vi "ADC SNR_Sweep - Copy.vi"(8 "error in (no error)":errorcluster, 9 "Sequence parameters":string[][](array[string])=[["Min limit", "Max limit", "Register sheet file", "Register Sheet"], ["", "", "CC2600.xls", "TX_BLE;Trim"], ["Reg write (addr;value)", "Operating frequency [Hz]", "", ""], ["NA", "2.44G", "", ""]], 10 "Run type":i32, 11 "Method parameters":T2={"Dev"={"Do not disturb DUT"=FALSE, "XOSC"=32000000.0, "Board type"="", "EM"="", "Configure tempboard"=TRUE, "Device specific info"=[], "Generic Object"=refnum}, "Method"={"Run type"=1, "Test name"="Current LPM2 4", "Comment"="", "Results folder"="", "AFC"=enum."Off", "Method name"="Current LPM2 4", "Method results"={"Excel brief report"=FALSE, "Spotfire report"=FALSE, "Starfish report"=FALSE}, "Operator"="", "Reference time"=timestamp(0 s since 1904-01-01), "AFC delay"=0.0, "Initialization"=enum."Enabled", "MD5 Sum"="", "HW addon board"=enum."None", "AFC Regsheet"="", "AFC Regfile"=path "", "dummy"=0.0}, "Inst"={"Instr"={"PS1"={"Name"="", "GPIB address"="", "VISA session"=""}, "PS2"={"Name"="", "GPIB address"="", "VISA session"=""}, "TC1"={"Name"="", "GPIB address"="", "VISA session"=""}, "TC2"={"Name"="", "GPIB address"="", "VISA session"=""}, "SA1"={"Name"="", "GPIB address"="", "VISA session"=""}, "SA2"={"Name"="", "GPIB address"="", "VISA session"=""}, "SG1"={"Name"="", "GPIB address"="", "VISA session"=""}, "SG2"={"Name"="", "GPIB address"="", "VISA session"=""}, "SG3"={"Name"="", "GPIB address"="", "VISA session"=""}, "MI1"={"Name"="", "GPIB address"="", "VISA session"=""}, "MI2"={"Name"="", "GPIB address"="", "VISA session"=""}, "SW SA"={"Name"="", "Controller addr"=""}, "SW SG"={"Name"="", "Controller addr"=""}, "MI3"={"Name"="", "GPIB address"="", "VISA session"=""}}, "Switchbox"={"RF Path"=0, "Cal compensation"=enum."TX", "Switchbox gain mode"="", "State"=enum."TX"}, "Instr to control (i.e. SA1)"="Default", "Intrument info string"=""}, "Sequence parameters"=[["Weight", "Min Limit", "Max Limit", "Register Sheet", "", "", "", "", "", "", "", "", ""], ["Vital", "", "1", "LPM2", "", "", "", "", "", "", "", "", ""], ["Resolution", "Reg write (addr;value)", "Chip mode", "Range", "", "", "", "", "", "", "", "", ""], ["u", "NA", "", "auto", "", "", "", "", "", "", "", "", ""]], "Cond"={"Temp logged"=25.0, "VDD1_PS1_6V"=-999.0, "VDD2_PS1_25V"=-999.0, "VDD4_PS2_25V"=-999.0, "VDD3_PS2_6V"=-999.0}, "Meas config"={"X-axis inner loop index"=32000000, "Y-axis outer loop index"=32000000, "X-axis"=[], "Y-axis"=[], "X-axis array req size"=32000000, "Y-axis array req size"=32000000, "Param description"=[], "Use meas clust for reporting"=FALSE, "Parameter index (page)"=0, "X-axis name"="", "Y-axis name"=""}} {"Cond"."VDD3_PS2_6V" format="%.3f"; "Cond"."VDD4_PS2_25V" format="%.3f"; "Cond"."VDD2_PS1_25V" format="%.3f"; "Cond"."VDD1_PS1_6V" format="%.3f"; "Method"."dummy" format="%.1p"; "Method"."AFC delay" format="%.1p"; "Dev"."XOSC" format="%.3p"}) -> (0 "Error Out":errorcluster[](array[cluster]), 1 "End Method Error":T2[](array[typedef]) {"Cond"."VDD3_PS2_6V" format="%.3f"; "Cond"."VDD4_PS2_25V" format="%.3f"; "Cond"."VDD2_PS1_25V" format="%.3f"; "Cond"."VDD1_PS1_6V" format="%.3f"; "Method"."dummy" format="%.1p"; "Method"."AFC delay" format="%.1p"; "Dev"."XOSC" format="%.3p"}, 2 "Short Results":string[](array[string]), 3 "Result summary":string[][](array[string])=[["Critical", "Output Power@2405 MHz", "-3", "4", "dBm"], ["Critical", "Output Power@2410 MHz", "-3", "4", "dBm"]])   [LabVIEW 2019]
doc: "[AutoDocStart]Performs crystal accuracy measurements. Measures the offset from ideal frequency. Primarily used for tuning XOSC capacitors and verifying XOSC trims.\n\nSweeping parameters: operating frequency, OSC override value and VDDR level\n\nResults: Offset frequency in ppm[AutoDocEnd]"
uses:
  User Lib/Utilities/Cluster definitions/Method input.ctl
  User Lib/Utilities/Cluster definitions/Device specific info.ctl
  User Lib/Utilities/Controls/Automatic Frequency Compensation types.ctl
  User Lib/Utilities/Controls/Method Reports.ctl
  User Lib/Utilities/Cluster definitions/Method Initialization.ctl
  User Lib/Utilities/Controls/HW addon boards.ctl
  User Lib/Utilities/Cluster definitions/Instr clust.ctl
  User Lib/Utilities/Switchbox control/SwitchBox_State._ENUMctl.ctl
  User Lib/Utilities/Cluster definitions/DUT vdd control.ctl
  User Lib/Utilities/Cluster definitions/DUT VDD4.ctl
  User Lib/Utilities/Cluster definitions/DUT VDD3.ctl
  User Lib/Utilities/Cluster definitions/DUT VDD2.ctl
  User Lib/Utilities/Cluster definitions/DUT VDD1.ctl
  User Lib/Generic chip methods/Classes/Generic_EM/Chameleon/Loki/Loki.lvclass
  69b5c8be-48d6-4f50-bcce-2a9f07fdba1a.vi
  1131283d-b54a-4ae3-ad67-71ff8f51acfe.vi
  3aacce8f-890b-4d9f-8ed2-28f84894822b.vi
  b456e919-2776-4fbb-a2ba-e4feed106c64.vi
  <vilib>/Utility/error.llb/Clear Errors.vi
  User Lib/Generic chip methods/Classes/Generic_EM/Chameleon/65nm.lvclass
  C:/Kharon/User Lib/Generic chip methods/Classes/Generic_EM/Generic_EM/Generic_EM.lvclass
  User Lib/Generic chip methods/board_to_chip_type.vi
  User Lib/Generic chip methods/Classes/Get_Class_init.vi
  User Lib/Generic chip methods/Classes/Generic_EM/Generic_EM/Generic_EM.lvclass
panel:
  out "Output Response [All DUTs] 7":u32[][](array[numeric])
  out "Dynamic Parameters 4":T1={"SNR"=nan, "SNRD"=nan, "THD"=nan, "ENOB (SNRD)"=nan, "SFDR"=nan, "ENOB (SNR)"=nan, "Noise Power"=nan, "Signal power"=nan} {"Signal power" format="%.6f"; "Noise Power" format="%.2f"; "ENOB (SNR)" format="%.2f"; "SFDR" format="%.2f"; "ENOB (SNRD)" format="%.2f"; "THD" format="%.2f"; "SNRD" format="%.2f"; "SNR" format="%.2f"}
  out "detected Throughput":dbl=200065.4236150998
  out "Output Response [All DUTs] 6":u32[][](array[numeric])
  out "Dynamic Parameters 3":T1={"SNR"=nan, "SNRD"=nan, "THD"=nan, "ENOB (SNRD)"=nan, "SFDR"=nan, "ENOB (SNR)"=nan, "Noise Power"=nan, "Signal power"=nan} {"Signal power" format="%.6f"; "Noise Power" format="%.2f"; "ENOB (SNR)" format="%.2f"; "SFDR" format="%.2f"; "ENOB (SNRD)" format="%.2f"; "THD" format="%.2f"; "SNRD" format="%.2f"; "SNR" format="%.2f"}
  out "detected Throughput":dbl=200065.4236150998
  out "Output Response [All DUTs] 5":u32[][](array[numeric])
  out "Dynamic Parameters 2":T1={"SNR"=nan, "SNRD"=nan, "THD"=nan, "ENOB (SNRD)"=nan, "SFDR"=nan, "ENOB (SNR)"=nan, "Noise Power"=nan, "Signal power"=nan} {"Signal power" format="%.6f"; "Noise Power" format="%.2f"; "ENOB (SNR)" format="%.2f"; "SFDR" format="%.2f"; "ENOB (SNRD)" format="%.2f"; "THD" format="%.2f"; "SNRD" format="%.2f"; "SNR" format="%.2f"}
  out "detected Throughput":dbl=200065.4236150998
  out "detected Throughput":dbl=200065.4236150998
  out "Dynamic Parameters":T1={"SNR"=nan, "SNRD"=nan, "THD"=nan, "ENOB (SNRD)"=nan, "SFDR"=nan, "ENOB (SNR)"=nan, "Noise Power"=nan, "Signal power"=nan} {"Signal power" format="%.6f"; "Noise Power" format="%.2f"; "ENOB (SNR)" format="%.2f"; "SFDR" format="%.2f"; "ENOB (SNRD)" format="%.2f"; "THD" format="%.2f"; "SNRD" format="%.2f"; "SNR" format="%.2f"}
  out "Output Response [All DUTs] 4":u32[][](array[numeric])
  in  "Tab Control":T10(tab)
  # "°C"
  # "°C"
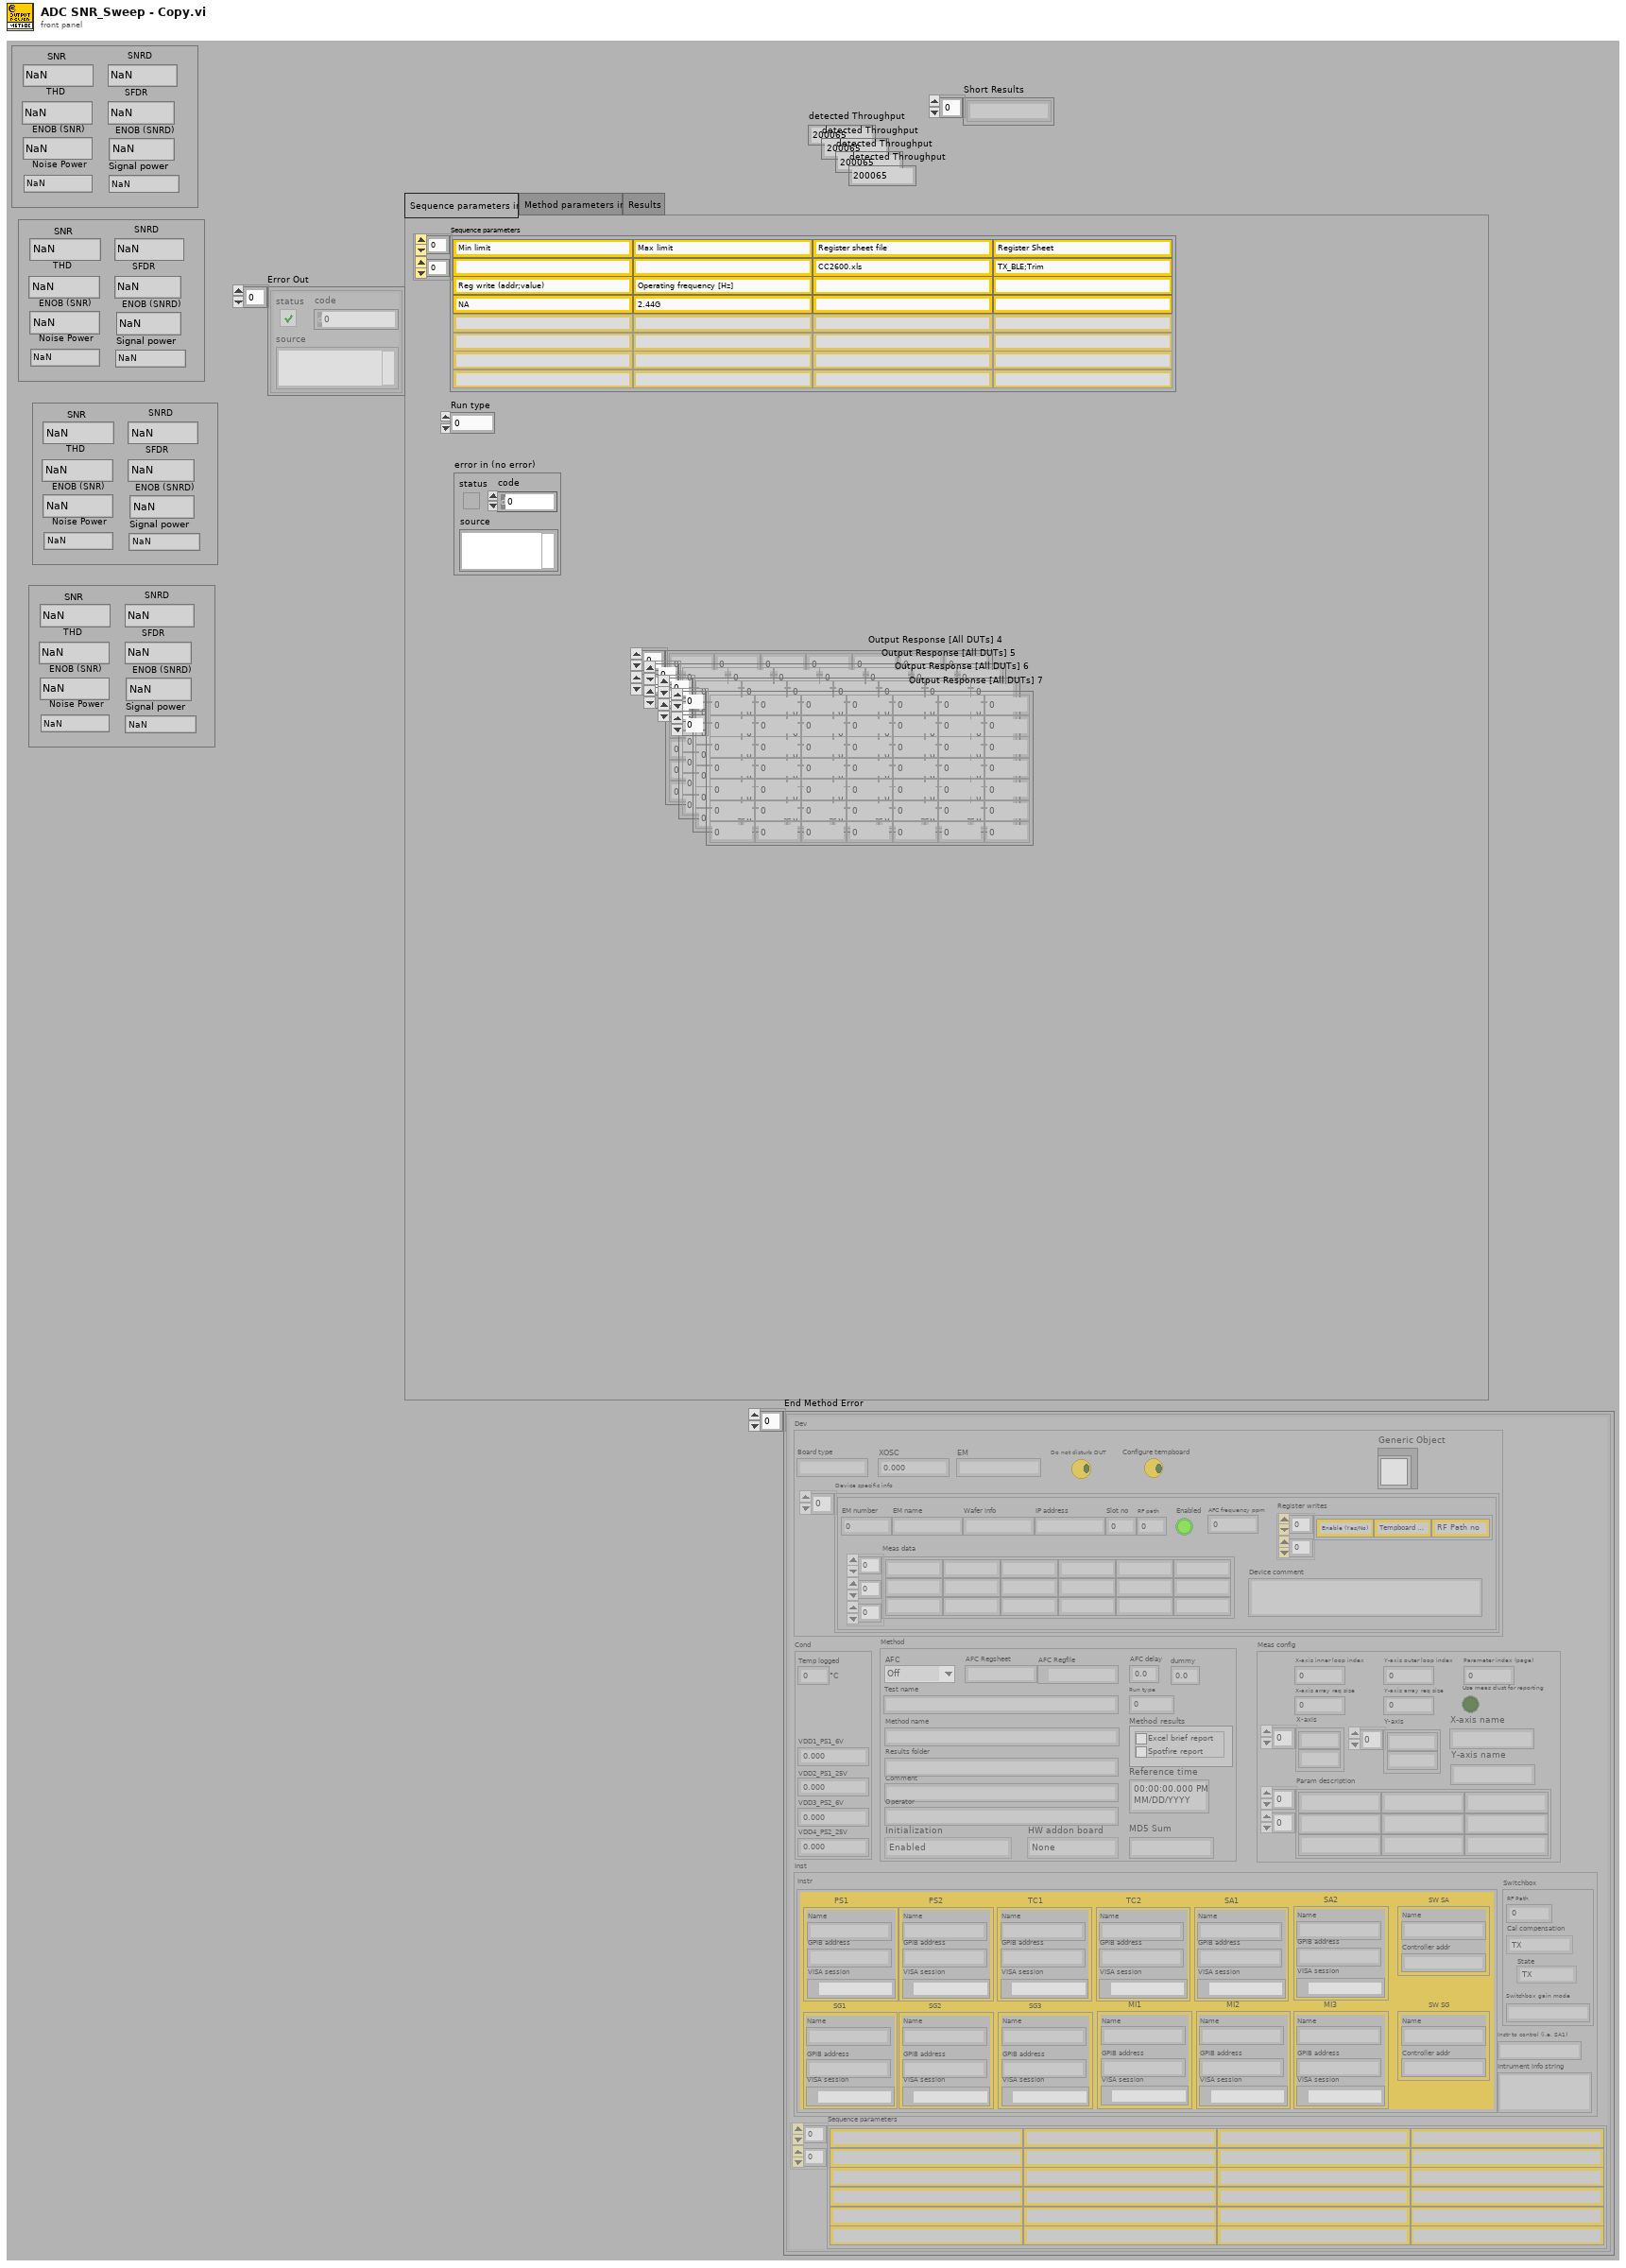
[diagram p1: front panel]
types:
  T1 = cluster{"SNR":dbl, "SNRD":dbl, "THD":dbl, "ENOB (SNRD)":dbl, "SFDR":dbl, "ENOB (SNR)":dbl, "Noise Power":dbl, "Signal power":dbl}
  T2 = typedef "Method input.ctl" = cluster{"Dev":cluster{"Do not disturb DUT":bool, "XOSC":dbl, "Board type":string, "EM":string, "Configure tempboard":bool, "Device specific info":T3[], "Generic Object":refnum<class>}, "Method":cluster{"Run type":i32, "Test name":string, "Comment":string, "Results folder":string, "AFC":T4, "Method name":string, "Method results":T5, "Operator":string, "Reference time":timestamp, "AFC delay":dbl, "Initialization":T6, "MD5 Sum":string, "HW addon board":T7, "AFC Regsheet":string, "AFC Regfile":path, "dummy":dbl}, "Inst":T8, "Sequence parameters":string[][], "Cond":cluster{"Temp logged":dbl, "VDD1_PS1_6V":dbl, "VDD2_PS1_25V":dbl, "VDD4_PS2_25V":dbl, "VDD3_PS2_6V":dbl}, "Meas config":cluster{"X-axis inner loop index":i32, "Y-axis outer loop index":i32, "X-axis":string[], "Y-axis":string[], "X-axis array req size":i32, "Y-axis array req size":i32, "Param description":string[][], "Use meas clust for reporting":bool, "Parameter index (page)":i32, "X-axis name":string, "Y-axis name":string}}
  T3 = typedef "Device specific info.ctl" = cluster{"EM number":u8, "IP address":string, "Enabled":bool, "Slot no":u8, "RF path":u8, "EM name":string, "Wafer info":string, "AFC frequency ppm":dbl, "Register writes":string[][], "Meas data":string[][][], "Device comment":string}
  T4 = typedef "Automatic Frequency Compensation types.ctl" = enum16{"Off", "Compensate Instrument frequency", "Compensate DUT frequency", "Predictive - Compensate Instrument frequency", "Predictive - Compensate DUT frequency", "Do not skip re-init - Compensate Instrument frequency", "Do not skip re-init - Compensate DUT frequency"}
  T5 = typedef "Method Reports.ctl" = cluster{"Excel brief report":bool, "Spotfire report":bool, "Starfish report":bool}
  T6 = typedef "Method Initialization.ctl" = enum16{"Enabled", "Skip Instr and Device Init", "Enabled with Separate Flash", "Set PS, Device Init and Skip Instr Init", "Skip Device Init"}
  T7 = typedef "HW addon boards.ctl" = enum16{"None", "Current meas 5EM", "Stresstest 10EM"}
  T8 = typedef "Instr clust.ctl" = cluster{"Instr":cluster{"PS1":cluster{"Name":string, "GPIB address":string, "VISA session":refnum<visa-resource-name>}, "PS2":cluster{"Name":string, "GPIB address":string, "VISA session":refnum<visa-resource-name>}, "TC1":cluster{"Name":string, "GPIB address":string, "VISA session":refnum<visa-resource-name>}, "TC2":cluster{"Name":string, "GPIB address":string, "VISA session":refnum<visa-resource-name>}, "SA1":cluster{"Name":string, "GPIB address":string, "VISA session":refnum<visa-resource-name>}, "SA2":cluster{"Name":string, "GPIB address":string, "VISA session":refnum<visa-resource-name>}, "SG1":cluster{"Name":string, "GPIB address":string, "VISA session":refnum<visa-resource-name>}, "SG2":cluster{"Name":string, "GPIB address":string, "VISA session":refnum<visa-resource-name>}, "SG3":cluster{"Name":string, "GPIB address":string, "VISA session":refnum<visa-resource-name>}, "MI1":cluster{"Name":string, "GPIB address":string, "VISA session":refnum<visa-resource-name>}, "MI2":cluster{"Name":string, "GPIB address":string, "VISA session":refnum<visa-resource-name>}, "SW SA":cluster{"Name":string, "Controller addr":string}, "SW SG":cluster{"Name":string, "Controller addr":string}, "MI3":cluster{"Name":string, "GPIB address":string, "VISA session":refnum<visa-resource-name>}}, "Switchbox":cluster{"RF Path":i32, "Cal compensation":enum16{"TX", "RX", "Interferer", "No compensation", "Interferer2"}, "Switchbox gain mode":string, "State":T9}, "Instr to control (i.e. SA1)":string, "Intrument info string":string}
  T9 = typedef "SwitchBox_State._ENUMctl.ctl" = enum16{"TX", "RX", "SP:TX", "SP:RX", "SW:TX", "SW:RX"}
  T10 = enum32{"Sequence parameters in", "Method parameters in", "Results"}
  T11 = typedef "DUT vdd control.ctl" = cluster{"VDD4 config":T12, "VDD3 config":T13, "VDD2 config":T14, "VDD1 config":T15}
  T12 = typedef "DUT VDD4.ctl" = u16
  T13 = typedef "DUT VDD3.ctl" = u16
  T14 = typedef "DUT VDD2.ctl" = u16
  T15 = typedef "DUT VDD1.ctl" = u16
  T16 = cluster{"Fundamental Frequency":dbl, "Sampling Frequncy":dbl, "No of Harmonics":u8, "Window":enum16{"None ", "Hanning", "Hamming", "Blackman-Harris", "Exact Blackman", "Blackman", "Flat Top", "4 Term B-Harris ", "7 Term B-Harris"}, "Blackman (fundamental power) bins)":dbl}
  T17 = enum32{"NI Card Settings", "Memory Read Setting", "DC Capture", "ADC Ramp", "ADC Sine", "SNR", "Cap Calibration"}
  T18 = enum32{"Read from Memory", "Read .dat file", "NI Card Capture", "None"}
  T19 = typedef "TFW ResponseData.ctl" = cluster{"errorCode":u32, "executionTime":u32, "processedCmdWord":u32, "responsePar":u32[], "actionCode":u32, "cmdStatus":u16}
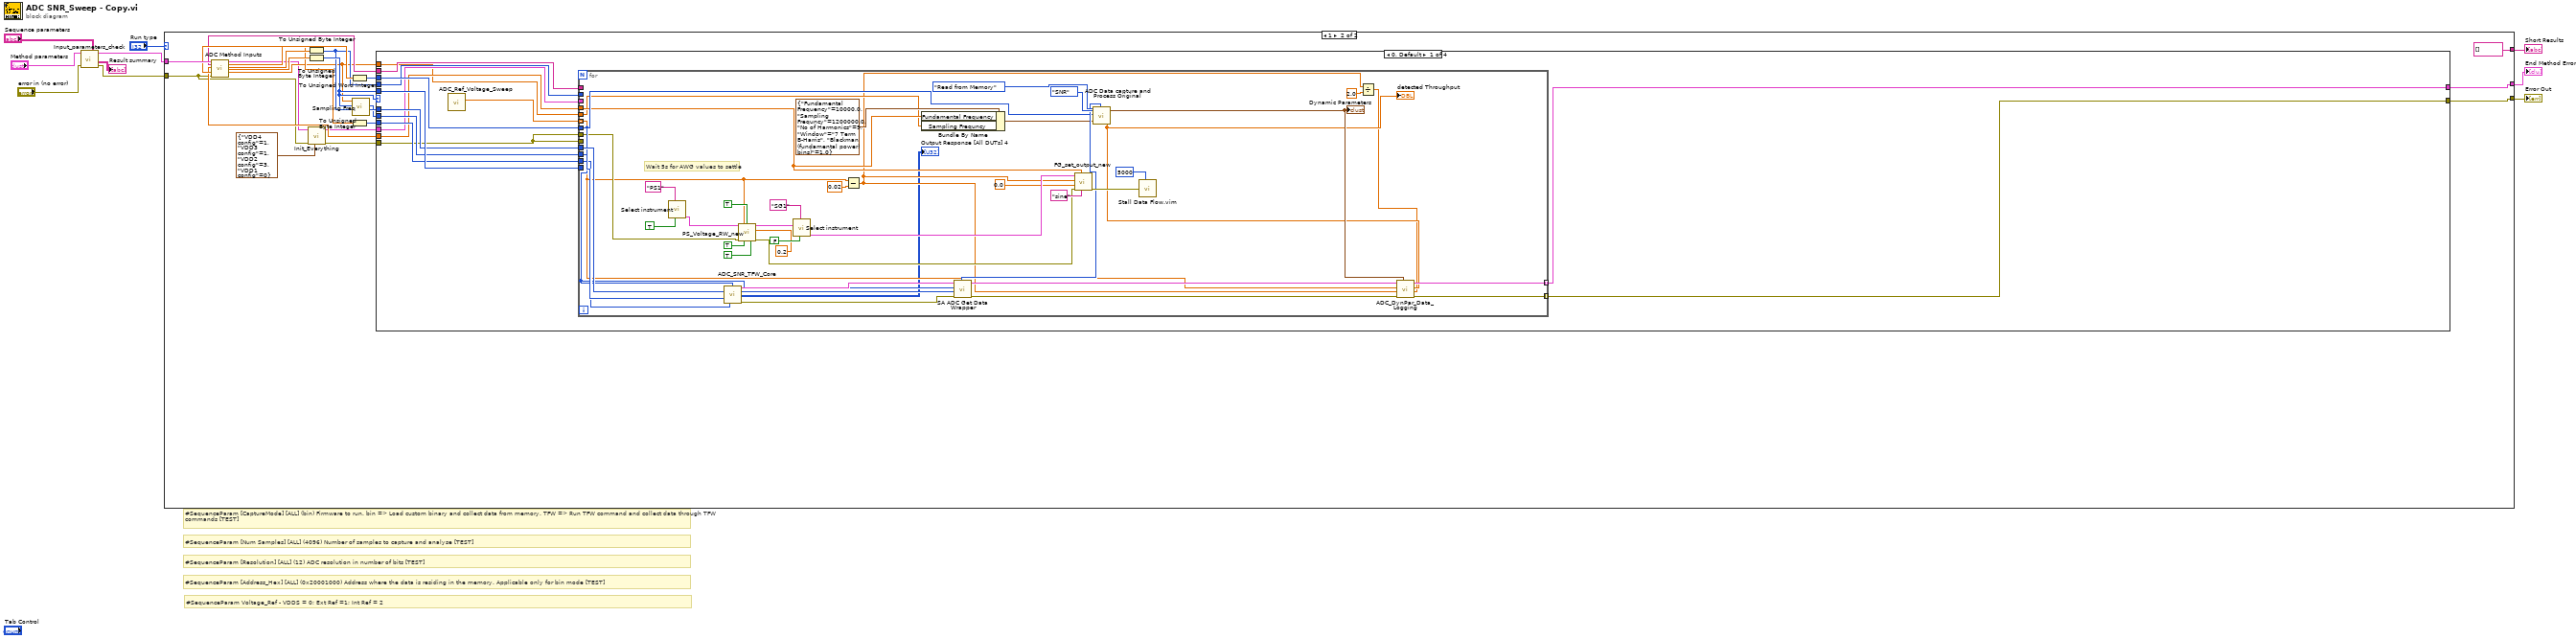
[diagram p0: block diagram]
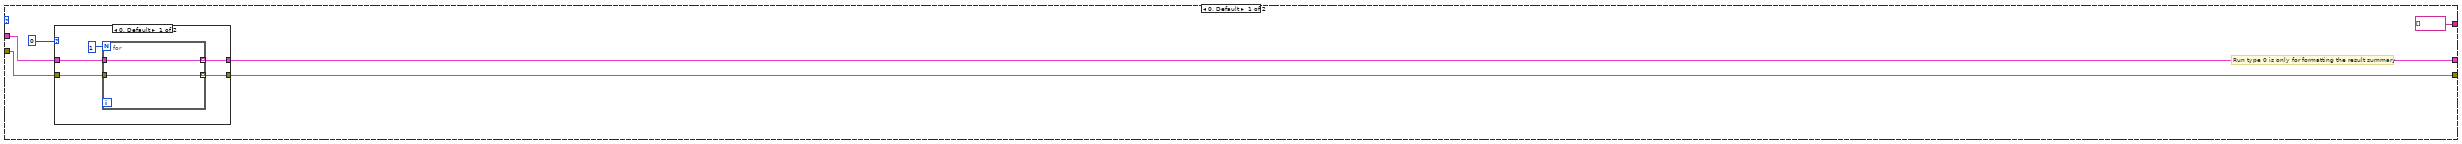
[diagram p2: hidden frame]
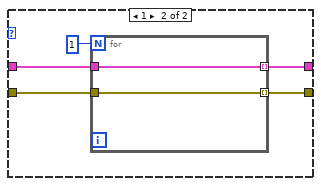
[diagram p3: hidden frame]
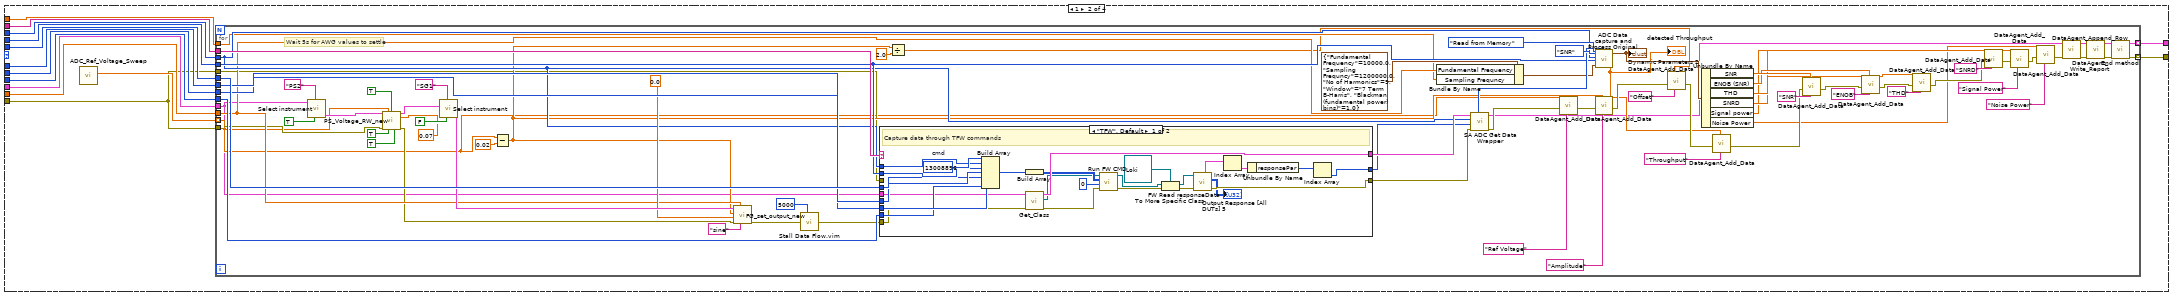
[diagram p4: hidden frame]
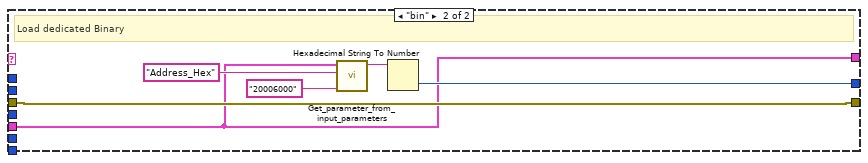
[diagram p5: hidden frame]
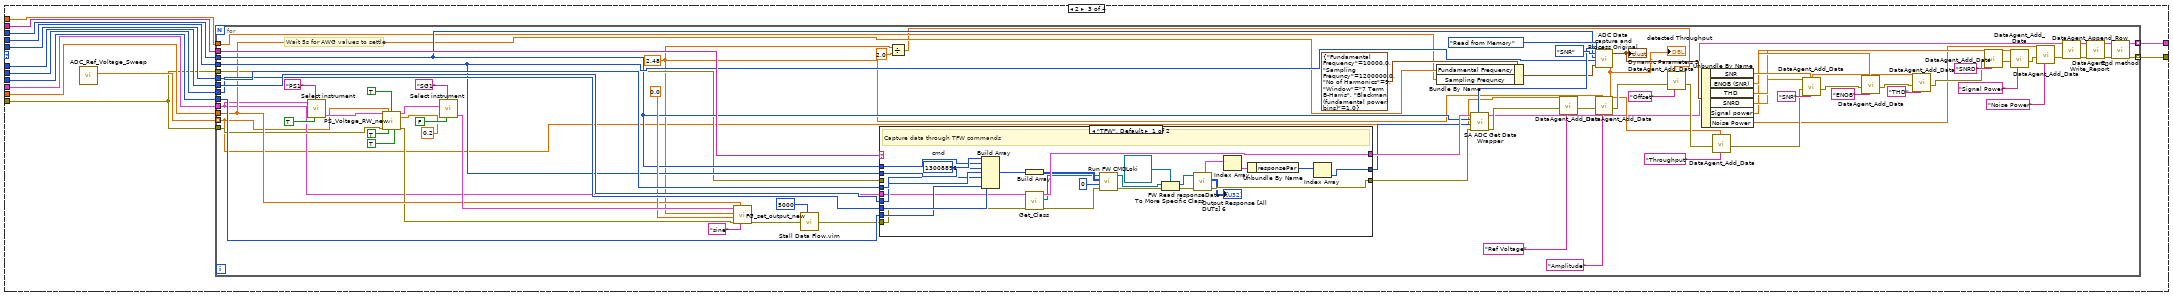
[diagram p6: hidden frame]
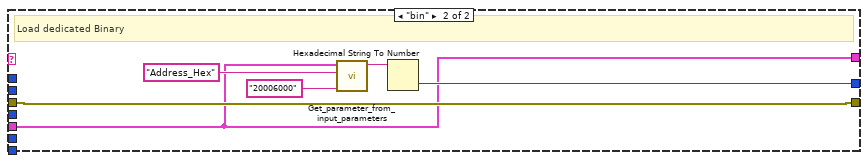
[diagram p7: hidden frame]
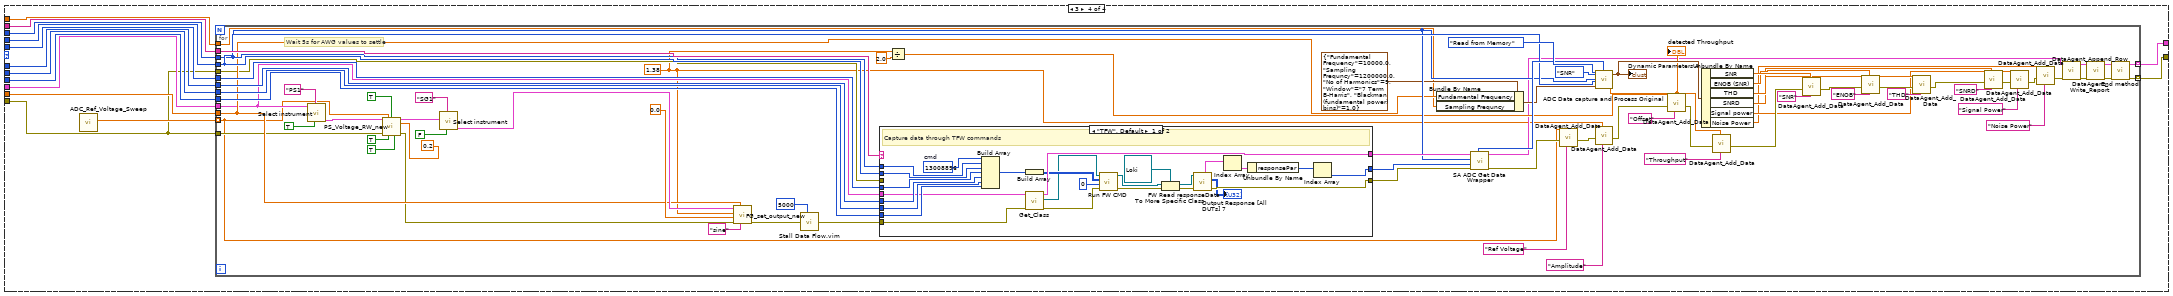
[diagram p8: hidden frame]
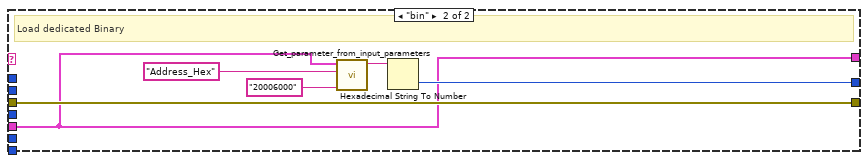
[diagram p9: hidden frame]
diagram:
  # "#SequenceParam Voltage_Ref - VDDS = 0; Ext Ref =1; Int Ref = 2"
  # "#SequenceParam [Num Samples] [ALL] (4096) Number of samples to capture and analyse [TEST]"
  # "#SequenceParam [CaptureMode] [ALL] (bin) Firmware to run. bin => Load custom binary and collect data from memory. TFW => Run TFW command and collect data through TFW commands [TEST]"
  # "#SequenceParam [Address_Hex] [ALL] (0x20001000) Address where the data is residing in the memory. Applicable only for bin mode [TEST]"
  # "#SequenceParam [Resolution] [ALL] (12) ADC resolution in number of bits [TEST]"
  n1 = call "Input_parameters_check.vi"("Sequence parameters"="Sequence parameters", "error in"="error in (no error)", "Method cluster in"="Method parameters") -> ("error out"=w10:errorcluster, "Result summary"=→"Result summary":string[][], "Method cluster out"=w6:T2)  [unwired: 6 in]
  n2 = case shown="1" "Run type" {
    tunnel: w10 -> [w12 w36]
    tunnel: w6 -> [w13 w52]
    tunnel: [w16 w38] -> w3
    tunnel: [w15 w37] -> w2
    tunnel: [string[] [] string[] []] -> w1
    frame 0, Default {
      # "Run type 0 is only for formatting the result summary"
      n3 = case shown="0, Default" 0 {
        tunnel: w13 -> [w21 w28]
        tunnel: w12 -> [w18 w27]
        tunnel: [w20 w26] -> w16
        tunnel: [w19 w25] -> w15
        frame 0, Default {
          n4 = for {
            N: 1 -> [_]
            tunnel: w21 -> [w23]
            tunnel: [w23] -> w20 mode=indexing
            tunnel: [w22] -> w19 mode=indexing
            tunnel: w18 -> [w22]
          }
        }
        frame 1 {
          n5 = for {
            N: 1 -> [_]
            tunnel: w28 -> [w30]
            tunnel: w27 -> [w29]
            tunnel: [w30] -> w26 mode=indexing
            tunnel: [w29] -> w25 mode=indexing
          }
        }
      }
    }
    frame 1 {
      n6 = call "ADC Method Inputs.vi"("Method cluster in"=w52, "error in (no error)"=w36) -> ("Capture Mode"=w40:string, "Signal Freq"=w43:dbl, "ADC Channel No."=w48:dbl, "Method cluster out"=w35:T2, "Num Samples"=w51:dbl, "Resolution"=w50:dbl, "Voltage Ref"=w49:dbl, "Sampling Freq"=w39:dbl)  [unwired: 6 in, 4 out]
      n7 = To Unsigned Byte Integer(number=w50) -> (unsigned 8bit integer=w41:u8)
      n8 = To Unsigned Byte Integer(number=w49) -> (unsigned 8bit integer=w42:u8)
      n9 = call "Init_Everything.vi"("VDD config"=T11 {"VDD4 config"=1, "VDD3 config"=1, "VDD2 config"=3, "VDD1 config"=0}, "error in"=w36, "Method cluster In"=w35) -> ("error out"=w33:errorcluster, "Method cluster out"=w34:T2)  [unwired: 5 in, 2 out]
      n10 = To Unsigned Word Integer(number=w51) -> (unsigned 16bit integer=w47:u16)
      n11 = To Unsigned Byte Integer(number=w48) -> (unsigned 8bit integer=w44:u8)
      n12 = call "Sampling Freq.vi"("Resolution"=w41, "Voltage Ref"=w42, "Sampling Freq"=w39) -> ("LGPT Count"=w46:u16, "SCOMP"=w45:u16)  [unwired: 7 in]
      n13 = case shown="0, Default" w42 {
        tunnel: w47 -> [w66 w123 w247 w370]
        tunnel: w41 -> [w65 w122 w246 w369]
        tunnel: w42 -> [w64 w121 w245 w368]
        tunnel: w46 -> [w63 w120 w244 w367]
        tunnel: w45 -> [w62 w119 w243 w366]
        tunnel: w44 -> [w61 w118 w242 w365]
        tunnel: w34 -> [w59 w116 w240 w363]
        tunnel: w33 -> [w53 w110 w234 w357]
        tunnel: w43 -> [w58 w115 w239 w362]
        tunnel: w40 -> [w57 w114 w238 w361]
        tunnel: w39 -> [w56 w113 w237 w360]
        tunnel: [w55 w112 w236 w359] -> w37
        tunnel: [w54 w111 w235 w358] -> w38
        frame 0, Default {
          n14 = call "ADC_Ref_Voltage_Sweep.vi"() -> ("Ref voltage sweep"=w60:dbl[])  [unwired: 11 in]
          n15 = for {
            tunnel: w66 -> [w90]
            tunnel: w65 -> [_]
            tunnel: w64 -> [_]
            tunnel: w63 -> [w106]
            tunnel: w62 -> [w105]
            tunnel: w61 -> [w104]
            tunnel: w57 -> [_]
            tunnel: w60 -> [w68] mode=indexing
            tunnel: w59 -> [_]
            tunnel: w53 -> [w80]
            tunnel: w58 -> [w87]
            tunnel: w56 -> [w86]
            tunnel: [w82] -> w55 mode=indexing
            tunnel: [w81] -> w54 mode=indexing
            tunnel: w53 -> [_]
            # "Wait 5s for AWG values to settle"
            n16 = call "Select instrument.vi"("Method cluster (T) / Instr cluster (F)"=TRUE, "Instr.Instr to control (i.e. SA1)"="PS1") -> ("Instr out"=w77:T8)  [unwired: 7 in, 2 out]
            n17 = call "ADC_SNR_TFW_Core.vi"("LGPT Count"=w90, "No. Samples"=w106, "Voltage Ref"=w105, "ADC Chnl No."=w104) -> ("Method cluster out 2"=w109:T2, "ResPar[0] Data Address"=w107:u32, "Output Response [All DUTs] 4"=→"Output Response [All DUTs] 4":u32[][], "error out"=w108:errorcluster)  [unwired: 8 in]
            n18 = call "PS_Voltage_RW_new.vi"("InstrCluster in"=w77, "Set Voltage"=w68, "Limit to 4V (T)"=TRUE, "Current(0)"=0.2, "error in (no error)"=w80, "Off (F)                         On (T)"=TRUE, "Read (F)                      Write (T)"=TRUE) -> ("InstrCluster out"=w78:T8, "error out"=w79:errorcluster)  [unwired: 6 in, 1 out]
            n19 = call "Select instrument.vi"("Method cluster (T) / Instr cluster (F)"=FALSE, "Instr.Instr to control (i.e. SA1)"="SG1", "Instr in"=w78) -> ("Instr out"=w98:T8)  [unwired: 6 in, 2 out]
            n20 = Subtract(x=w68, y=0.02) -> (x-y=w69:dbl)
            n21 = Bundle By Name(cluster=T16 {"Fundamental Frequency"=10000.0, "Sampling Frequncy"=1200000.0, "No of Harmonics"=9, "Window"=enum."7 Term B-Harris", "Blackman (fundamental power) bins)"=1.0} ("Inputs for Dyanmic para"), "Fundamental Frequency"=w87, "Sampling Frequncy"=w86) -> (w88:T16)
            n22 = call "SA ADC Get Data Wrapper.vi"("error in"=w108, "Data Address"=w107, "Num Samples"=w90, "Method cluster in"=w109) -> ("error out"=w83:errorcluster, "output cluster"=w72:T2, "Output in mV"=w91:u32[])  [unwired: 2 in, 3 out]
            n23 = call "FG_set_output_new.vi"("Function (DC, Sine, Square, Triangle, Ramp up, Ramp down, Pulse)"="sine", "Frequency [Hz]"=w87, "error in"=w79, "Low voltage"=0.0, "High voltage (or DC)"=w69, "InstrCluster in"=w98) -> ("error out"=w95:errorcluster)  [unwired: 4 in, 1 out]
            n24 = call "ADC Data capture and Process Original.vi"("ADC Output Read Method"=T18."Read from Memory", "Select the Tab to project"=T17."SNR", "No.of samples(SNR)"=w90, "Inputs for Dyanmic para"=w88, "Waveform"=w91) -> ("detected Throughput"=w71:dbl, "Dynamic Parameters"=w85:T1)  [unwired: 16 in, 5 out]
            "Dynamic Parameters" <- w85
            "detected Throughput" <- w71
            n25 = call "Stall Data Flow.vim"("value in"=w95, "milliseconds to wait"=u32 5000) -> ()  [unwired: 2 out]
            n26 = Divide(x=w69, y=2.0) -> (x/y=w70:dbl)
            n27 = call "ADC_DynPar_Data_Logging.vi"("Offset (V)"=w70, "detected Throughput"=w71, "Dynamic Parameters"=w85, "error in (no error)"=w83, "Amplitude (Vpp)"=w69, "Ref Voltage"=w68, "Method Cluster In"=w72) -> ("error out"=w82:errorcluster, "Method cluster out"=w81:T2)  [unwired: 3 in]
          }
        }
        frame 1 {
          n28 = call "ADC_Ref_Voltage_Sweep.vi"() -> ("Ref voltage sweep"=w117:dbl[])  [unwired: 11 in]
          n29 = for {
            tunnel: w123 -> [w178]
            tunnel: w122 -> [w179]
            tunnel: w121 -> [w198]
            tunnel: w120 -> [w197]
            tunnel: w119 -> [w196]
            tunnel: w118 -> [w195]
            tunnel: w114 -> [w194]
            tunnel: w117 -> [w127] mode=indexing
            tunnel: w116 -> [w125]
            tunnel: w110 -> [w133]
            tunnel: w115 -> [w175]
            tunnel: w113 -> [w174]
            tunnel: [w136] -> w112 mode=indexing
            tunnel: [w135] -> w111 mode=indexing
            tunnel: w110 -> [w134]
            # "Wait 5s for AWG values to settle"
            n30 = call "Select instrument.vi"("Method cluster (T) / Instr cluster (F)"=TRUE, "Instr.Instr to control (i.e. SA1)"="PS2", "Method cluster in"=w125) -> ("Instr out"=w130:T8)  [unwired: 6 in, 2 out]
            n31 = call "PS_Voltage_RW_new.vi"("InstrCluster in"=w130, "Set Voltage"=w127, "Limit to 4V (T)"=TRUE, "Current(0)"=0.07, "error in (no error)"=w133, "Off (F)                         On (T)"=TRUE, "Read (F)                      Write (T)"=TRUE) -> ("InstrCluster out"=w131:T8, "error out"=w132:errorcluster)  [unwired: 6 in, 1 out]
            n32 = call "Select instrument.vi"("Method cluster (T) / Instr cluster (F)"=FALSE, "Instr.Instr to control (i.e. SA1)"="SG1", "Instr in"=w131) -> ("Instr out"=w188:T8)  [unwired: 6 in, 2 out]
            n33 = Subtract(x=w127, y=0.02) -> (x-y=w155:dbl)
            n34 = call "FG_set_output_new.vi"("Function (DC, Sine, Square, Triangle, Ramp up, Ramp down, Pulse)"="sine", "Frequency [Hz]"=w175, "error in"=w132, "Low voltage"=0.0, "High voltage (or DC)"=w155, "InstrCluster in"=w188) -> ("error out"=w185:errorcluster)  [unwired: 4 in, 1 out]
            n35 = call "Stall Data Flow.vim"("value in"=w185, "milliseconds to wait"=u32 5000) -> ("value out"=w184:errorcluster)  [unwired: 1 out]
            n36 = case shown="\"TFW\", Default" w194 {
              tunnel: [w227 w228] -> w201
              tunnel: [w222 w229] -> w200
              tunnel: [w210 w230] -> w199
              tunnel: w178 -> [w209 _]
              tunnel: w179 -> [w208 _]
              tunnel: w198 -> [w207 _]
              tunnel: w197 -> [w206 _]
              tunnel: w196 -> [w205 _]
              tunnel: w195 -> [w204 _]
              tunnel: w125 -> [w203 w228]
              tunnel: w184 -> [w202 _]
              tunnel: w134 -> [_ w229]
              frame "TFW", Default {
                w225 = u32 13008896  # cmd
                # "Capture data through TFW commands"
                n37 = Build Array(w225, w209, w208, w207, w206, w205, w204) -> (w224:u32[])
                n38 = Build Array(w224) -> (w223:u32[][])
                n39 = call "Get_Class.vi"("error in (no error)"=w202, "Method cluster in"=w203) -> ("error out"=w220:errorcluster, "Class Out"=w219:refnum<class "Generic_EM.lvclass">, "Method cluster out"=w227:T2)  [unwired: 6 in, 1 out]
                n40 = call-dynamic "Run FW CMD.vi"("error in (no error)"=w220, "Handler"=u8 0, "cmdBuf"=w223, "Generic_EM in"=w219) -> ("error out"=w215:errorcluster, "Generic_EM out"=w218:refnum<class "Generic_EM.lvclass">)  [unwired: 6 in]
                n41 = To More Specific Class(target class=refnum<class "Loki.lvclass"> refnum ("Loki in"), reference=w218, error in=w215) -> (specific class reference=w216:refnum<class "Loki.lvclass">, error out=w214:errorcluster)
                n42 = call "FW Read responseData.vi"("error in (no error)"=w214, "Loki in"=w216) -> ("error out"=w222:errorcluster, "Output Response [All DUTs]"=→"Output Response [All DUTs] 5":u32[][], "Response"=w212:T19[])  [unwired: 6 in, 1 out]
                n43 = Index Array(array=w212) -> (element=w213:T19)  [unwired: 1 in]
                n44 = Unbundle By Name(w213) -> ("responsePar"=w211:u32[])
                n45 = Index Array(array=w211) -> (element=w210:u32)  [unwired: 1 in]
              }
              frame "bin" {
                # "Load dedicated Binary"
                n46 = call "Get_parameter_from_input_parameters.vi"("Default value (used if not specified on Front Panel)"="20006000", "Parameter name"="Address_Hex" ("SA_ param name"), "Method cluster (if input param empty)"=w228) -> ("value as String"=w233:string)  [unwired: 2 in, 6 out]
                n47 = Hexadecimal String To Number(string=w233) -> (number=w230:u32)  [unwired: 2 in, 1 out]
              }
            }
            n48 = Divide(x=w155, y=2.0) -> (x/y=w153:dbl)
            n49 = Bundle By Name(cluster=T16 {"Fundamental Frequency"=10000.0, "Sampling Frequncy"=1200000.0, "No of Harmonics"=9, "Window"=enum."7 Term B-Harris", "Blackman (fundamental power) bins)"=1.0} ("Inputs for Dyanmic para"), "Fundamental Frequency"=w175, "Sampling Frequncy"=w174) -> (w176:T16)
            n50 = call "SA ADC Get Data Wrapper.vi"("error in"=w200, "Data Address"=w199, "Num Samples"=w178, "Method cluster in"=w201) -> ("error out"=w145:errorcluster, "output cluster"=w138:T2, "Output in mV"=w180:u32[])  [unwired: 2 in, 3 out]
            n51 = call "DataAgent_Add_Data.vi"("ColumnName"="Ref Voltage", "Data"=w127, "error in (no error)"=w145) -> ("error out"=w143:errorcluster)  [unwired: 8 in]
            n52 = call "ADC Data capture and Process Original.vi"("ADC Output Read Method"=T18."Read from Memory", "Select the Tab to project"=T17."SNR", "No.of samples(SNR)"=w178, "Resolution"=w179, "Inputs for Dyanmic para"=w176, "Waveform"=w180) -> ("detected Throughput"=w152:dbl, "Dynamic Parameters"=w173:T1)  [unwired: 15 in, 5 out]
            "Dynamic Parameters 2" <- w173
            "detected Throughput" <- w152
            n53 = call "DataAgent_Add_Data.vi"("ColumnName"="Amplitude" ("Default Value"), "Data"=w155, "error in (no error)"=w143) -> ("error out"=w171:errorcluster)  [unwired: 8 in]
            n54 = call "DataAgent_Add_Data.vi"("ColumnName"="Offset" ("Default Value"), "Data"=w153, "error in (no error)"=w171) -> ("error out"=w157:errorcluster)  [unwired: 8 in]
            n55 = Unbundle By Name(w173) -> ("SNR"=w151:dbl, "ENOB (SNR)"=w150:dbl, "THD"=w149:dbl, "SNRD"=w148:dbl, "Signal power"=w147:dbl, "Noise Power"=w146:dbl)
            n56 = call "DataAgent_Add_Data.vi"("ColumnName"="Throughput", "Data"=w152, "error in (no error)"=w157) -> ("error out"=w156:errorcluster)  [unwired: 8 in]
            n57 = call "DataAgent_Add_Data.vi"("ColumnName"="SNR", "Data"=w151, "error in (no error)"=w156) -> ("error out"=w169:errorcluster)  [unwired: 8 in]
            n58 = call "DataAgent_Add_Data.vi"("ColumnName"="ENOB", "Data"=w150, "error in (no error)"=w169) -> ("error out"=w164:errorcluster)  [unwired: 8 in]
            n59 = call "DataAgent_Add_Data.vi"("ColumnName"="THD", "Data"=w149, "error in (no error)"=w164) -> ("error out"=w163:errorcluster)  [unwired: 8 in]
            n60 = call "DataAgent_Add_Data.vi"("ColumnName"="SNRD", "Data"=w148, "error in (no error)"=w163) -> ("error out"=w162:errorcluster)  [unwired: 8 in]
            n61 = call "DataAgent_Add_Data.vi"("ColumnName"="Signal Power", "Data"=w147, "error in (no error)"=w162) -> ("error out"=w159:errorcluster)  [unwired: 8 in]
            n62 = call "DataAgent_Add_Data.vi"("ColumnName"="Noise Power", "Data"=w146, "error in (no error)"=w159) -> ("error out"=w137:errorcluster)  [unwired: 8 in]
            n63 = call "DataAgent_Append_Row.vi"("error in (no error)"=w137, "Method cluster in"=w138) -> ("error out"=w139:errorcluster, "Method cluster out"=w140:T2)  [unwired: 8 in]
            n64 = call "DataAgent_Write_Report.vi"("error in (no error)"=w139, "Method cluster in"=w140) -> ("error out"=w142:errorcluster, "Method cluster out"=w141:T2)  [unwired: 8 in]
            n65 = call "End method.vi"("error in"=w142, "Method cluster in"=w141) -> ("error out"=w136:errorcluster, "Method cluster out"=w135:T2)  [unwired: 7 in, 1 out]
          }
        }
        frame 2 {
          n66 = call "ADC_Ref_Voltage_Sweep.vi"() -> ("Ref voltage sweep"=w241:dbl[])  [unwired: 11 in]
          n67 = for {
            tunnel: w247 -> [w302]
            tunnel: w246 -> [w303]
            tunnel: w245 -> [w321]
            tunnel: w244 -> [w320]
            tunnel: w243 -> [w319]
            tunnel: w242 -> [w318]
            tunnel: w238 -> [w317]
            tunnel: w241 -> [w249] mode=indexing
            tunnel: w240 -> [w251]
            tunnel: w234 -> [w258]
            tunnel: w239 -> [w299]
            tunnel: w237 -> [w298]
            tunnel: [w261] -> w236 mode=indexing
            tunnel: [w260] -> w235 mode=indexing
            tunnel: w234 -> [w259]
            w250 = 2.48 ("High voltage (or DC)")
            # "Wait 5s for AWG values to settle"
            n68 = call "Select instrument.vi"("Method cluster (T) / Instr cluster (F)"=TRUE, "Instr.Instr to control (i.e. SA1)"="PS1", "Method cluster in"=w251) -> ("Instr out"=w255:T8)  [unwired: 6 in, 2 out]
            n69 = call "PS_Voltage_RW_new.vi"("InstrCluster in"=w255, "Set Voltage"=w249, "Limit to 4V (T)"=TRUE, "Current(0)"=0.2, "error in (no error)"=w258, "Off (F)                         On (T)"=TRUE, "Read (F)                      Write (T)"=TRUE) -> ("InstrCluster out"=w256:T8, "error out"=w257:errorcluster)  [unwired: 6 in, 1 out]
            n70 = call "Select instrument.vi"("Method cluster (T) / Instr cluster (F)"=FALSE, "Instr.Instr to control (i.e. SA1)"="SG1", "Instr in"=w256) -> ("Instr out"=w312:T8)  [unwired: 6 in, 2 out]
            n71 = call "FG_set_output_new.vi"("Function (DC, Sine, Square, Triangle, Ramp up, Ramp down, Pulse)"="sine", "Frequency [Hz]"=w299, "error in"=w257, "Low voltage"=0.0, "High voltage (or DC)"=w250, "InstrCluster in"=w312) -> ("error out"=w309:errorcluster)  [unwired: 4 in, 1 out]
            n72 = call "Stall Data Flow.vim"("value in"=w309, "milliseconds to wait"=u32 5000) -> ("value out"=w308:errorcluster)  [unwired: 1 out]
            n73 = case shown="\"TFW\", Default" w317 {
              tunnel: [w350 w351] -> w324
              tunnel: [w345 w352] -> w323
              tunnel: [w333 w353] -> w322
              tunnel: w302 -> [w332 _]
              tunnel: w303 -> [w331 _]
              tunnel: w321 -> [w330 _]
              tunnel: w320 -> [w329 _]
              tunnel: w319 -> [w328 _]
              tunnel: w318 -> [w327 _]
              tunnel: w251 -> [w326 w351]
              tunnel: w308 -> [w325 _]
              tunnel: w259 -> [_ w352]
              frame "TFW", Default {
                w348 = u32 13008896  # cmd
                # "Capture data through TFW commands"
                n74 = Build Array(w348, w332, w331, w330, w329, w328, w327) -> (w347:u32[])
                n75 = Build Array(w347) -> (w346:u32[][])
                n76 = call "Get_Class.vi"("error in (no error)"=w325, "Method cluster in"=w326) -> ("error out"=w343:errorcluster, "Class Out"=w342:refnum<class "Generic_EM.lvclass">, "Method cluster out"=w350:T2)  [unwired: 6 in, 1 out]
                n77 = call-dynamic "Run FW CMD.vi"("error in (no error)"=w343, "Handler"=u8 0, "cmdBuf"=w346, "Generic_EM in"=w342) -> ("error out"=w338:errorcluster, "Generic_EM out"=w341:refnum<class "Generic_EM.lvclass">)  [unwired: 6 in]
                n78 = To More Specific Class(target class=refnum<class "Loki.lvclass"> refnum ("Loki in"), reference=w341, error in=w338) -> (specific class reference=w339:refnum<class "Loki.lvclass">, error out=w337:errorcluster)
                n79 = call "FW Read responseData.vi"("error in (no error)"=w337, "Loki in"=w339) -> ("error out"=w345:errorcluster, "Output Response [All DUTs]"=→"Output Response [All DUTs] 6":u32[][], "Response"=w335:T19[])  [unwired: 6 in, 1 out]
                n80 = Index Array(array=w335) -> (element=w336:T19)  [unwired: 1 in]
                n81 = Unbundle By Name(w336) -> ("responsePar"=w334:u32[])
                n82 = Index Array(array=w334) -> (element=w333:u32)  [unwired: 1 in]
              }
              frame "bin" {
                # "Load dedicated Binary"
                n83 = call "Get_parameter_from_input_parameters.vi"("Default value (used if not specified on Front Panel)"="20006000", "Parameter name"="Address_Hex" ("SA_ param name"), "Method cluster (if input param empty)"=w351) -> ("value as String"=w356:string)  [unwired: 2 in, 6 out]
                n84 = Hexadecimal String To Number(string=w356) -> (number=w353:u32)  [unwired: 2 in, 1 out]
              }
            }
            n85 = Divide(x=w250, y=2.0) -> (x/y=w278:dbl)
            n86 = Bundle By Name(cluster=T16 {"Fundamental Frequency"=10000.0, "Sampling Frequncy"=1200000.0, "No of Harmonics"=9, "Window"=enum."7 Term B-Harris", "Blackman (fundamental power) bins)"=1.0} ("Inputs for Dyanmic para"), "Fundamental Frequency"=w299, "Sampling Frequncy"=w298) -> (w300:T16)
            n87 = call "SA ADC Get Data Wrapper.vi"("error in"=w323, "Data Address"=w322, "Num Samples"=w302, "Method cluster in"=w324) -> ("error out"=w270:errorcluster, "output cluster"=w263:T2, "Output in mV"=w304:u32[])  [unwired: 2 in, 3 out]
            n88 = call "DataAgent_Add_Data.vi"("ColumnName"="Ref Voltage", "Data"=w249, "error in (no error)"=w270) -> ("error out"=w268:errorcluster)  [unwired: 8 in]
            n89 = call "ADC Data capture and Process Original.vi"("ADC Output Read Method"=T18."Read from Memory", "Select the Tab to project"=T17."SNR", "No.of samples(SNR)"=w302, "Resolution"=w303, "Inputs for Dyanmic para"=w300, "Waveform"=w304) -> ("detected Throughput"=w277:dbl, "Dynamic Parameters"=w297:T1)  [unwired: 15 in, 5 out]
            "Dynamic Parameters 3" <- w297
            "detected Throughput" <- w277
            n90 = call "DataAgent_Add_Data.vi"("ColumnName"="Amplitude" ("Default Value"), "Data"=w250, "error in (no error)"=w268) -> ("error out"=w295:errorcluster)  [unwired: 8 in]
            n91 = call "DataAgent_Add_Data.vi"("ColumnName"="Offset" ("Default Value"), "Data"=w278, "error in (no error)"=w295) -> ("error out"=w281:errorcluster)  [unwired: 8 in]
            n92 = Unbundle By Name(w297) -> ("SNR"=w276:dbl, "ENOB (SNR)"=w275:dbl, "THD"=w274:dbl, "SNRD"=w273:dbl, "Signal power"=w272:dbl, "Noise Power"=w271:dbl)
            n93 = call "DataAgent_Add_Data.vi"("ColumnName"="Throughput", "Data"=w277, "error in (no error)"=w281) -> ("error out"=w280:errorcluster)  [unwired: 8 in]
            n94 = call "DataAgent_Add_Data.vi"("ColumnName"="SNR", "Data"=w276, "error in (no error)"=w280) -> ("error out"=w293:errorcluster)  [unwired: 8 in]
            n95 = call "DataAgent_Add_Data.vi"("ColumnName"="ENOB", "Data"=w275, "error in (no error)"=w293) -> ("error out"=w288:errorcluster)  [unwired: 8 in]
            n96 = call "DataAgent_Add_Data.vi"("ColumnName"="THD", "Data"=w274, "error in (no error)"=w288) -> ("error out"=w287:errorcluster)  [unwired: 8 in]
            n97 = call "DataAgent_Add_Data.vi"("ColumnName"="SNRD", "Data"=w273, "error in (no error)"=w287) -> ("error out"=w286:errorcluster)  [unwired: 8 in]
            n98 = call "DataAgent_Add_Data.vi"("ColumnName"="Signal Power", "Data"=w272, "error in (no error)"=w286) -> ("error out"=w283:errorcluster)  [unwired: 8 in]
            n99 = call "DataAgent_Add_Data.vi"("ColumnName"="Noise Power", "Data"=w271, "error in (no error)"=w283) -> ("error out"=w262:errorcluster)  [unwired: 8 in]
            n100 = call "DataAgent_Append_Row.vi"("error in (no error)"=w262, "Method cluster in"=w263) -> ("error out"=w264:errorcluster, "Method cluster out"=w265:T2)  [unwired: 8 in]
            n101 = call "DataAgent_Write_Report.vi"("error in (no error)"=w264, "Method cluster in"=w265) -> ("error out"=w267:errorcluster, "Method cluster out"=w266:T2)  [unwired: 8 in]
            n102 = call "End method.vi"("error in"=w267, "Method cluster in"=w266) -> ("error out"=w261:errorcluster, "Method cluster out"=w260:T2)  [unwired: 7 in, 1 out]
          }
        }
        frame 3 {
          n103 = call "ADC_Ref_Voltage_Sweep.vi"() -> ("Ref voltage sweep"=w364:dbl[])  [unwired: 11 in]
          n104 = for {
            tunnel: w370 -> [w425]
            tunnel: w369 -> [w426]
            tunnel: w368 -> [w444]
            tunnel: w367 -> [w443]
            tunnel: w366 -> [w442]
            tunnel: w365 -> [w441]
            tunnel: w361 -> [w440]
            tunnel: w364 -> [w372] mode=indexing
            tunnel: w363 -> [w374]
            tunnel: w357 -> [w381]
            tunnel: w362 -> [w422]
            tunnel: w360 -> [w421]
            tunnel: [w384] -> w359 mode=indexing
            tunnel: [w383] -> w358 mode=indexing
            tunnel: w357 -> [w382]
            w373 = 1.38 ("High voltage (or DC)")
            # "Wait 5s for AWG values to settle"
            n105 = call "Select instrument.vi"("Method cluster (T) / Instr cluster (F)"=TRUE, "Instr.Instr to control (i.e. SA1)"="PS1", "Method cluster in"=w374) -> ("Instr out"=w378:T8)  [unwired: 6 in, 2 out]
            n106 = call "PS_Voltage_RW_new.vi"("InstrCluster in"=w378, "Set Voltage"=w372, "Limit to 4V (T)"=TRUE, "Current(0)"=0.2, "error in (no error)"=w381, "Off (F)                         On (T)"=TRUE, "Read (F)                      Write (T)"=TRUE) -> ("InstrCluster out"=w379:T8, "error out"=w380:errorcluster)  [unwired: 6 in, 1 out]
            n107 = call "Select instrument.vi"("Method cluster (T) / Instr cluster (F)"=FALSE, "Instr.Instr to control (i.e. SA1)"="SG1", "Instr in"=w379) -> ("Instr out"=w435:T8)  [unwired: 6 in, 2 out]
            n108 = call "FG_set_output_new.vi"("Function (DC, Sine, Square, Triangle, Ramp up, Ramp down, Pulse)"="sine", "Frequency [Hz]"=w422, "error in"=w380, "Low voltage"=0.0, "High voltage (or DC)"=w373, "InstrCluster in"=w435) -> ("error out"=w432:errorcluster)  [unwired: 4 in, 1 out]
            n109 = call "Stall Data Flow.vim"("value in"=w432, "milliseconds to wait"=u32 5000) -> ("value out"=w431:errorcluster)  [unwired: 1 out]
            n110 = case shown="\"TFW\", Default" w440 {
              tunnel: [w473 w474] -> w447
              tunnel: [w468 w475] -> w446
              tunnel: [w456 w476] -> w445
              tunnel: w425 -> [w455 _]
              tunnel: w426 -> [w454 _]
              tunnel: w444 -> [w453 _]
              tunnel: w443 -> [w452 _]
              tunnel: w442 -> [w451 _]
              tunnel: w441 -> [w450 _]
              tunnel: w374 -> [w449 w474]
              tunnel: w431 -> [w448 _]
              tunnel: w382 -> [_ w475]
              frame "TFW", Default {
                w471 = u32 13008896  # cmd
                # "Capture data through TFW commands"
                n111 = Build Array(w471, w455, w454, w453, w452, w451, w450) -> (w470:u32[])
                n112 = Build Array(w470) -> (w469:u32[][])
                n113 = call "Get_Class.vi"("error in (no error)"=w448, "Method cluster in"=w449) -> ("error out"=w466:errorcluster, "Class Out"=w465:refnum<class "Generic_EM.lvclass">, "Method cluster out"=w473:T2)  [unwired: 6 in, 1 out]
                n114 = call-dynamic "Run FW CMD.vi"("error in (no error)"=w466, "Handler"=u8 0, "cmdBuf"=w469, "Generic_EM in"=w465) -> ("error out"=w461:errorcluster, "Generic_EM out"=w464:refnum<class "Generic_EM.lvclass">)  [unwired: 6 in]
                n115 = To More Specific Class(target class=refnum<class "Loki.lvclass"> refnum ("Loki in"), reference=w464, error in=w461) -> (specific class reference=w462:refnum<class "Loki.lvclass">, error out=w460:errorcluster)
                n116 = call "FW Read responseData.vi"("error in (no error)"=w460, "Loki in"=w462) -> ("error out"=w468:errorcluster, "Output Response [All DUTs]"=→"Output Response [All DUTs] 7":u32[][], "Response"=w458:T19[])  [unwired: 6 in, 1 out]
                n117 = Index Array(array=w458) -> (element=w459:T19)  [unwired: 1 in]
                n118 = Unbundle By Name(w459) -> ("responsePar"=w457:u32[])
                n119 = Index Array(array=w457) -> (element=w456:u32)  [unwired: 1 in]
              }
              frame "bin" {
                # "Load dedicated Binary"
                n120 = call "Get_parameter_from_input_parameters.vi"("Default value (used if not specified on Front Panel)"="20006000", "Parameter name"="Address_Hex" ("SA_ param name"), "Method cluster (if input param empty)"=w474) -> ("value as String"=w479:string)  [unwired: 2 in, 6 out]
                n121 = Hexadecimal String To Number(string=w479) -> (number=w476:u32)  [unwired: 2 in, 1 out]
              }
            }
            n122 = Divide(x=w373, y=2.0) -> (x/y=w401:dbl)
            n123 = Bundle By Name(cluster=T16 {"Fundamental Frequency"=10000.0, "Sampling Frequncy"=1200000.0, "No of Harmonics"=9, "Window"=enum."7 Term B-Harris", "Blackman (fundamental power) bins)"=1.0} ("Inputs for Dyanmic para"), "Fundamental Frequency"=w422, "Sampling Frequncy"=w421) -> (w423:T16)
            n124 = call "SA ADC Get Data Wrapper.vi"("error in"=w446, "Data Address"=w445, "Num Samples"=w425, "Method cluster in"=w447) -> ("error out"=w393:errorcluster, "output cluster"=w386:T2, "Output in mV"=w427:u32[])  [unwired: 2 in, 3 out]
            n125 = call "DataAgent_Add_Data.vi"("ColumnName"="Ref Voltage", "Data"=w372, "error in (no error)"=w393) -> ("error out"=w391:errorcluster)  [unwired: 8 in]
            n126 = call "ADC Data capture and Process Original.vi"("ADC Output Read Method"=T18."Read from Memory", "Select the Tab to project"=T17."SNR", "No.of samples(SNR)"=w425, "Resolution"=w426, "Inputs for Dyanmic para"=w423, "Waveform"=w427) -> ("detected Throughput"=w400:dbl, "Dynamic Parameters"=w420:T1)  [unwired: 15 in, 5 out]
            "Dynamic Parameters 4" <- w420
            "detected Throughput" <- w400
            n127 = call "DataAgent_Add_Data.vi"("ColumnName"="Amplitude" ("Default Value"), "Data"=w373, "error in (no error)"=w391) -> ("error out"=w418:errorcluster)  [unwired: 8 in]
            n128 = call "DataAgent_Add_Data.vi"("ColumnName"="Offset" ("Default Value"), "Data"=w401, "error in (no error)"=w418) -> ("error out"=w404:errorcluster)  [unwired: 8 in]
            n129 = Unbundle By Name(w420) -> ("SNR"=w399:dbl, "ENOB (SNR)"=w398:dbl, "THD"=w397:dbl, "SNRD"=w396:dbl, "Signal power"=w395:dbl, "Noise Power"=w394:dbl)
            n130 = call "DataAgent_Add_Data.vi"("ColumnName"="Throughput", "Data"=w400, "error in (no error)"=w404) -> ("error out"=w403:errorcluster)  [unwired: 8 in]
            n131 = call "DataAgent_Add_Data.vi"("ColumnName"="SNR", "Data"=w399, "error in (no error)"=w403) -> ("error out"=w416:errorcluster)  [unwired: 8 in]
            n132 = call "DataAgent_Add_Data.vi"("ColumnName"="ENOB", "Data"=w398, "error in (no error)"=w416) -> ("error out"=w411:errorcluster)  [unwired: 8 in]
            n133 = call "DataAgent_Add_Data.vi"("ColumnName"="THD", "Data"=w397, "error in (no error)"=w411) -> ("error out"=w410:errorcluster)  [unwired: 8 in]
            n134 = call "DataAgent_Add_Data.vi"("ColumnName"="SNRD", "Data"=w396, "error in (no error)"=w410) -> ("error out"=w409:errorcluster)  [unwired: 8 in]
            n135 = call "DataAgent_Add_Data.vi"("ColumnName"="Signal Power", "Data"=w395, "error in (no error)"=w409) -> ("error out"=w406:errorcluster)  [unwired: 8 in]
            n136 = call "DataAgent_Add_Data.vi"("ColumnName"="Noise Power", "Data"=w394, "error in (no error)"=w406) -> ("error out"=w385:errorcluster)  [unwired: 8 in]
            n137 = call "DataAgent_Append_Row.vi"("error in (no error)"=w385, "Method cluster in"=w386) -> ("error out"=w387:errorcluster, "Method cluster out"=w388:T2)  [unwired: 8 in]
            n138 = call "DataAgent_Write_Report.vi"("error in (no error)"=w387, "Method cluster in"=w388) -> ("error out"=w390:errorcluster, "Method cluster out"=w389:T2)  [unwired: 8 in]
            n139 = call "End method.vi"("error in"=w390, "Method cluster in"=w389) -> ("error out"=w384:errorcluster, "Method cluster out"=w383:T2)  [unwired: 7 in, 1 out]
          }
        }
      }
    }
  }
  "End Method Error" <- w3
  "Error Out" <- w2
  "Short Results" <- w1
